vi "UT_JSONLFormatter_Main.vi"(8 "error in":errorcluster) -> (0 "error out":errorcluster)   [LabVIEW 2016, in "UT_JSONLFormatter.lvlib"]
doc: "Collection of tests for JSONLFormatter class."
uses:
  UT_JSONLFormatter.lvlib
  <vilib>/addons/_JKI Toolkits/Caraya/classes/Test/Test.lvclass
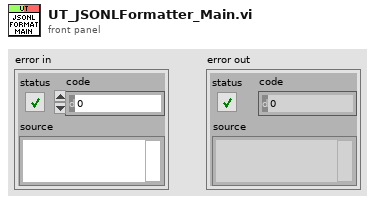
[diagram p1: front panel]
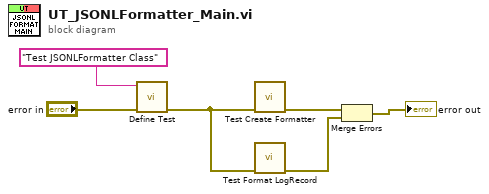
[diagram p0: block diagram]
diagram:
  n1 = call <vilib>:"Define Test.vi"("error in (no error)"="error in", "Label (VI Title)"="Test JSONLFormatter Class") -> ("error out"=w2:errorcluster)  [unwired: 8 in, 1 out]
  n2 = call "Test Create Formatter.vi"("error in"=w2) -> ("error out"=w4:errorcluster)  [unwired: 10 in]
  n3 = call "Test Format LogRecord.vi"("error in"=w2) -> ("error out"=w1:errorcluster)  [unwired: 10 in]
  n4 = Merge Errors(w4, w1) -> (→"error out":errorcluster)
